vi "自动-整理取料点补偿值数据.vi"(8 "取料对刀/复锁对刀":enum16{"取料补偿", "复锁补偿"}(ring), 9 "拧紧程式序号数组":i32[](array[numeric]), 10 "上视觉补偿机械手移动量 mm输入":T2 {"X" format="%#.3f"}, 11 "Img输入":T1) -> (2 "发送给PLC数据数组":dbl[](array[numeric]), 3 "机械手移动量 mm输出":T2 {"X" format="%#.3f"})   [LabVIEW 2014]
uses:
  Global.vi
  Controls/XYZRPos.ctl
  Controls/XYPos.ctl
  <vilib>/vision/Image Controls.llb/IMAQ Image.ctl
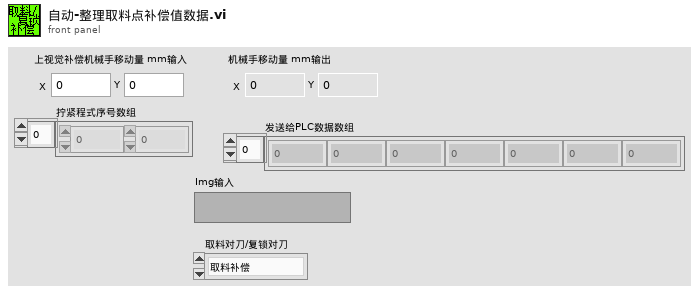
[diagram p1: front panel]
types:
  T1 = typedef "IMAQ Image.ctl" = refnum<image>
  T2 = typedef "XYPos.ctl" = cluster{"X":dbl, "Y":dbl}
  T3 = typedef "XYZRPos.ctl" = cluster{"X":dbl, "Y":dbl, "Z":dbl, "R":dbl}
  T4 = typedef "ModeEditeControl.ctl" = cluster{"AllModelFold":path, "AllModelNamePath":path, "所有零件型号":string[], "当前零件型号":string, "所有建立零件信息":string[][], "当前零件序号":i32, "当前产品信息":T5}
  T5 = typedef "ModelInfo.ctl" = cluster{"产品型号":string, "二维码拍照":u32, "Mark点拍照":u32}
  T6 = typedef "XYZRPos+左右手.ctl" = cluster{"坐标":T3, "左右手":dbl}
  T7 = cluster{"[0]":dbl, "[1]":dbl, "[2]":dbl, "[3]":dbl}
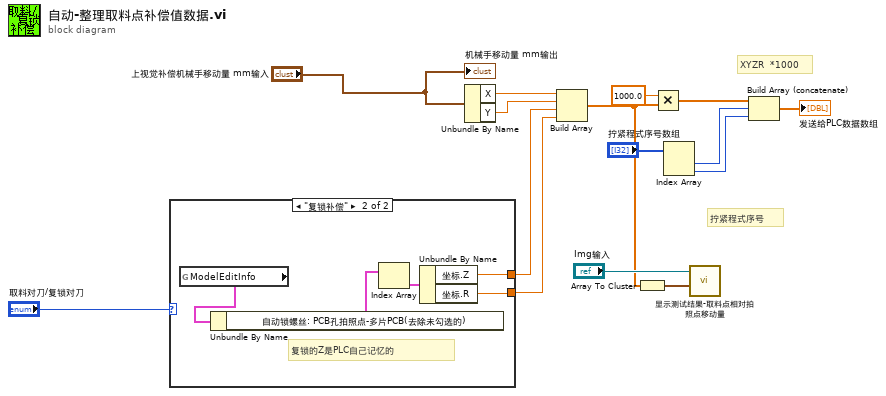
[diagram p0: block diagram]
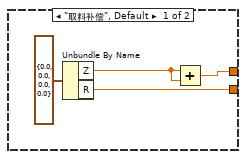
[diagram p2: hidden frame]
diagram:
  # "XYZR  *1000"
  # "拧紧程式序号"
  n1 = case shown="\"复锁补偿\"" "取料对刀/复锁对刀" {
    tunnel: [w19 w21] -> w10
    tunnel: [w18 w20] -> w9
    frame "取料补偿", Default {
      n2 = Unbundle By Name(T3 {"X"=0.0, "Y"=0.0, "Z"=0.0, "R"=0.0} ("输入簇")) -> ("Z"=w16:dbl, "R"=w18:dbl)
      n3 = Add(x=w16, y=w16) -> (x+y=w19:dbl)
    }
    frame "复锁补偿" {
      # "复锁的Z是PLC自己记忆的"
      n4 = global read "Global.vi" "ModelEditInfo"() -> (w24:T4)
      n5 = Unbundle By Name(w24) -> ("自动锁螺丝: PCB孔拍照点-多片PCB(去除未勾选的)"=w23:T6[])
      n6 = Index Array(array=w23) -> (element=w22:T6)  [unwired: 1 in]
      n7 = Unbundle By Name(w22) -> ("坐标.Z"=w21:dbl, "坐标.R"=w20:dbl)
    }
  }
  n8 = Unbundle By Name("上视觉补偿机械手移动量 mm输入") -> ("X"=w14:dbl, "Y"=w15:dbl)
  n9 = Build Array(w14, w15, w10, w9) -> (w3:dbl[])
  n10 = Array To Cluster(array=w3) -> (cluster=w4:T7)
  n11 = Multiply(x=1000.0, y=w3) -> (x*y=w13:dbl[])
  n12 = Index Array(array="拧紧程式序号数组") -> (element #1=w7:i32, element #2=w6:i32)  [unwired: 2 in]
  n13 = call "显示测试结果-取料点相对拍照点移动量.vi"("当前取料点(XY为需要再移动量，ZR为实际值)"=w4, "Img输入"="Img输入") -> ()  [unwired: 10 in]
  n14 = Build Array (concatenate)(w13, w7, w6) -> (→"发送给PLC数据数组":dbl[])
  "机械手移动量 mm输出" <- "上视觉补偿机械手移动量 mm输入"
